vi "Create Local Events.vi"() -> (0 "error out":errorcluster, 3 "Local Events":T1)   [LabVIEW 2020, in "Lock-in amplifier.lvlib" / "Local Events.lvlib"]
doc: "____\nPantherLAB Templates 1.0.0.5\nCopyright (c) 2022, PantherLAB"
uses:
  Local Events.lvlib
  Local Events--cluster.ctl
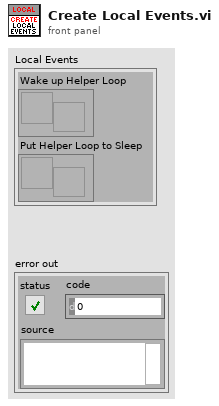
[diagram p1: front panel]
types:
  T1 = typedef "Lock-in amplifier.lvlib/Local Events.lvlib/Local Events--cluster.ctl" = cluster{"Wake up Helper Loop":refnum<user-event>, "Put Helper Loop to Sleep":refnum<user-event>}
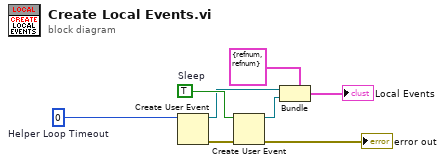
[diagram p0: block diagram]
diagram:
  w6 = TRUE  # Sleep
  w3 = 0  # Helper Loop Timeout
  n1 = Create User Event(user event datatype=w3) -> (user event=w4:refnum<user-event>, error out=w8:errorcluster)  [unwired: 1 in]
  n2 = Create User Event(user event datatype=w6, error in=w8) -> (user event=w5:refnum<user-event>, error out=→"error out":errorcluster)
  n3 = Bundle(cluster=T1 {"Wake up Helper Loop"=refnum, "Put Helper Loop to Sleep"=refnum} ("Local Events"), "Wake up Helper Loop"=w4, "Put Helper Loop to Sleep"=w5) -> (→"Local Events":T1)
